vi "Formic Princess.vi"(8 "error in (no error)":errorcluster, 9 "SelfID":i32, 10 "Map":i32[](array[numeric]), 11 "Mother in":refnum<class "Formics.lvclass">) -> (0 "error out":errorcluster, 1 "Direction":T1, 2 "Action":T2, 3 "Mother out":refnum<class "Formics.lvclass">, 4 "Replicated Class":refnum<class "Formics.lvclass">)   [LabVIEW 2015, in "Formics.lvclass"]
uses:
  Formics.lvclass
  Type Defs/Action Enum.ctl
  Type Defs/Direction Enum.ctl
  Formics.lvclass/Formics.ctl
  SquareStatus.ctl
  Formic Types.ctl
  Type Defs/SB Type Defs.lvlib
  Common/Common.lvlib
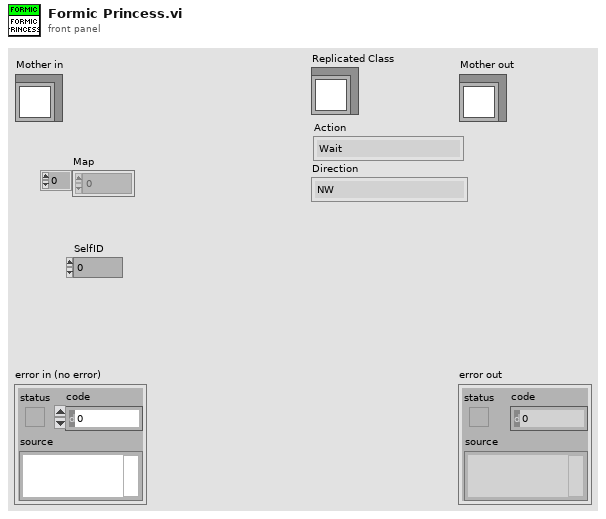
[diagram p1: front panel]
types:
  T1 = typedef "SB Type Defs.lvlib/Direction Enum.ctl" = enum16{"NW", "N", "NE", "E", "SE", "S", "SW", "W"}
  T2 = typedef "SB Type Defs.lvlib/Action Enum.ctl" = enum16{"Wait", "Move", "Attack", "Replicate"}
  T3 = typedef "Formics.lvclass/Formic Types.ctl" = enum16{"Queen Bee", "Protector Bee", "Daughter Bee", "Worker Bee", "Coward"}
  T4 = typedef "Formics.lvclass/SquareStatus.ctl" = cluster{"ID":i32, "Heartbeat":bool, "MyPosition":cluster{"X":i32, "Y":i32}}
  T5 = typedef "Formics.lvclass/SquareStatus DVR.ctl" = refnum<data-value>
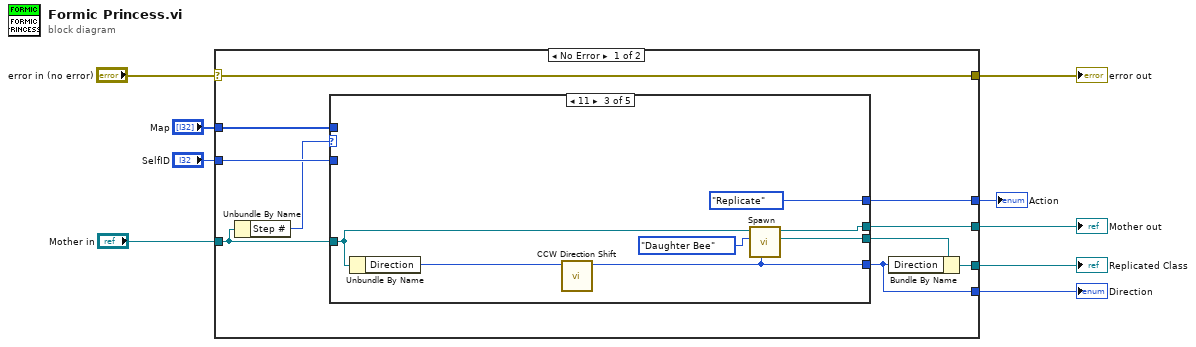
[diagram p0: block diagram]
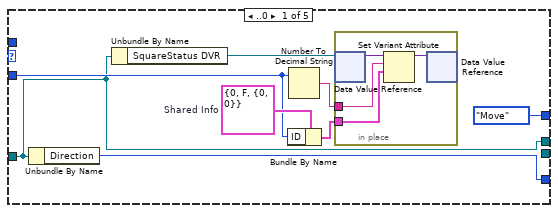
[diagram p2: hidden frame]
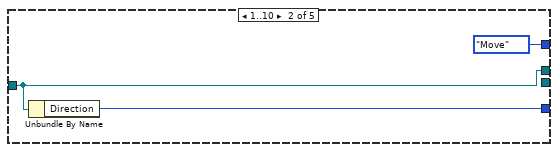
[diagram p3: hidden frame]
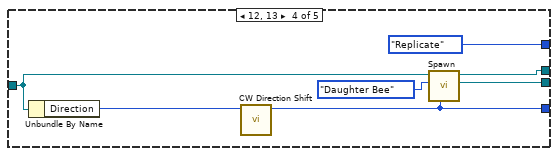
[diagram p4: hidden frame]
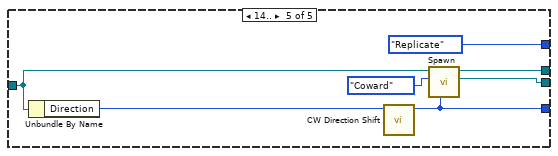
[diagram p5: hidden frame]
diagram:
  n1 = case shown="No Error" "error in (no error)" {
    selector: "error in (no error)" -> [w19 w57]
    tunnel: [w19 w57] -> w8
    tunnel: [w18 w56] -> w6
    tunnel: "Mother in" -> [w17 w56]
    tunnel: "SelfID" -> [w16 _]
    tunnel: "Map" -> [w15 _]
    tunnel: [w14 _] -> w3
    tunnel: [w12 _] -> w2
    tunnel: [w13 _] -> w1
    frame No Error {
      n2 = Unbundle By Name(w17) -> ("Step #"=w10:i32)
      n3 = case shown="11" w10 {
        tunnel: w17 -> [w21 w34 w37 w44 w51]
        tunnel: [w21 w34 w40 w47 w54] -> w18
        tunnel: w15 -> [_ _ _ _ _]
        tunnel: [Action_Enum."Move" ("Action") Action_Enum."Move" ("Action") Action_Enum."Replicate" ("Action") Action_Enum."Replicate" ("Action") Action_Enum."Replicate" ("Action")] -> w14
        tunnel: [w20 w32 w35 w42 w50] -> w12
        tunnel: [_ _ w39 w46 w53] -> w11
        tunnel: w16 -> [w23 _ _ _ _]
        frame ..0 {
          w26 = T4 {"ID"=0, "Heartbeat"=FALSE, "MyPosition"={"X"=0, "Y"=0}}  # Shared Info
          n4 = Unbundle By Name(w21) -> ("Direction"=w20:i32)
          n5 = Unbundle By Name(w21) -> ("SquareStatus DVR"=w27:T5)
          n6 = Bundle By Name(cluster=w26, "ID"=w23) -> (w24:T4)
          n7 = Number To Decimal String(number=w23) -> (decimal integer string=w25:string)  [unwired: 1 in]
          n8 = in-place {
            in-place-border: w25 -> [w29]
            in-place-border: w24 -> [w28]
            n9 = in-place-dvr #1(w27) -> (w31:variant)  [unwired: 1 out]
            n10 = Set Variant Attribute(Variant=w31, name=w29, value=w28) -> (Variant out=w30:variant)  [unwired: 1 in, 2 out]
            n11 = in-place-dvr #1(w30) -> ()  [unwired: 2 out]
          }
        }
        frame 1..10 {
          n12 = Unbundle By Name(w34) -> ("Direction"=w32:i32)
        }
        frame 11 {
          n13 = Unbundle By Name(w37) -> ("Direction"=w36:i32)
          n14 = call "CCW Direction Shift.vi"("Direction"=w36) -> ("Numeric"=w35:i32)  [unwired: 10 in]
          n15 = call "Spawn.vi"("Start Direction"=w35, "Directive"=Formic_Types."Daughter Bee", "Mother in"=w37) -> ("Replicated Class"=w39:refnum<class "Formics.lvclass">, "Mother out"=w40:refnum<class "Formics.lvclass">)  [unwired: 6 in, 1 out]
        }
        frame 12, 13 {
          n16 = Unbundle By Name(w44) -> ("Direction"=w43:i32)
          n17 = call "CW Direction Shift.vi"("Direction"=w43) -> ("Numeric"=w42:i32)  [unwired: 10 in]
          n18 = call "Spawn.vi"("Start Direction"=w42, "Directive"=Formic_Types."Daughter Bee", "Mother in"=w44) -> ("Replicated Class"=w46:refnum<class "Formics.lvclass">, "Mother out"=w47:refnum<class "Formics.lvclass">)  [unwired: 6 in, 1 out]
        }
        frame 14.. {
          n19 = Unbundle By Name(w51) -> ("Direction"=w49:i32)
          n20 = call "CW Direction Shift.vi"("Direction"=w49) -> ("Numeric"=w50:i32)  [unwired: 10 in]
          n21 = call "Spawn.vi"("Start Direction"=w50, "Directive"=Formic_Types."Coward", "Mother in"=w51) -> ("Replicated Class"=w53:refnum<class "Formics.lvclass">, "Mother out"=w54:refnum<class "Formics.lvclass">)  [unwired: 6 in, 1 out]
        }
      }
      n22 = Bundle By Name(cluster=w11, "Direction"=w12) -> (w13:refnum<class "Formics.lvclass">)
    }
    frame Error {
    }
  }
  "error out" <- w8
  "Mother out" <- w6
  "Action" <- w3
  "Direction" <- w2
  "Replicated Class" <- w1
